vi "printFunc_preLabelPrint_wmg.vi"(7 "时间标识":timestamp format="%<%y/%m/%d>T", 8 "路径":path, 9 "Data in":string[](array[string]), 10 "input_str_PN":string="1", 11 "VISA resource name":refnum<visa-resource-name>="USB0::0x0A5F::0x00AB::JJL045601::RAW") -> (0 "exsit":bool, 3 "条码输出":string)   [LabVIEW 2011]
uses:
  <vilib>/Utility/file.llb/Read From Spreadsheet File (string).vi
  <vilib>/Utility/file.llb/Write To Spreadsheet File (string).vi
panel:
  # "0. P/N  luxshare\n1. Product Type *\n2. AWG\n3. Length\n4. SN\n5. Rev\n6. Custmer PN \n7. Vendor Number *\n8. Location *\n9. Label Title *"
  # "P/N  luxshare"
  # "Product Type *"
  # "AWG"
  # "Length"
  # "SN"
  # "Rev"
  # "Customer"
  # "Vender Num *"
  # "Location *"
  # "Label Title *"
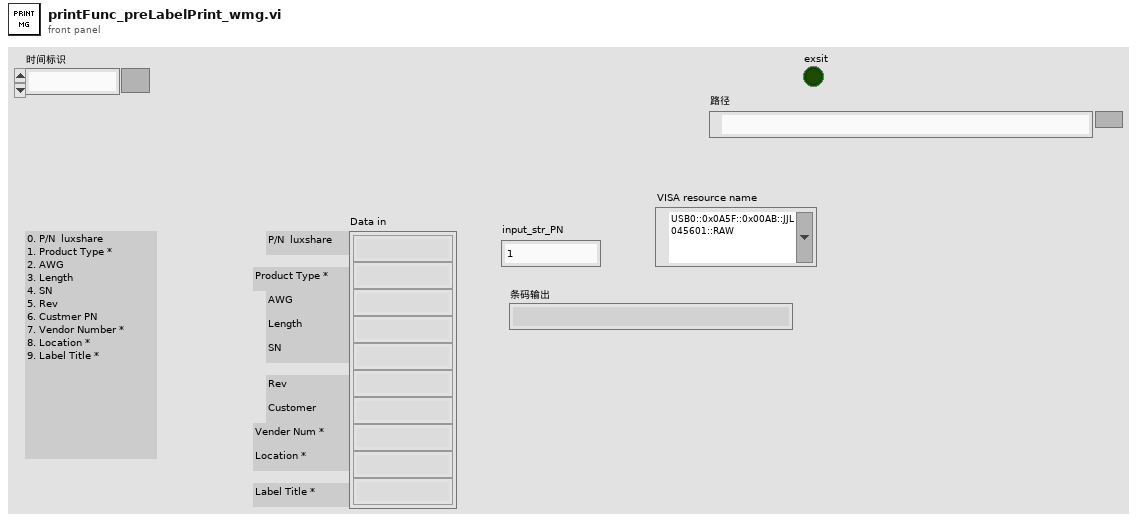
[diagram p1: front panel]
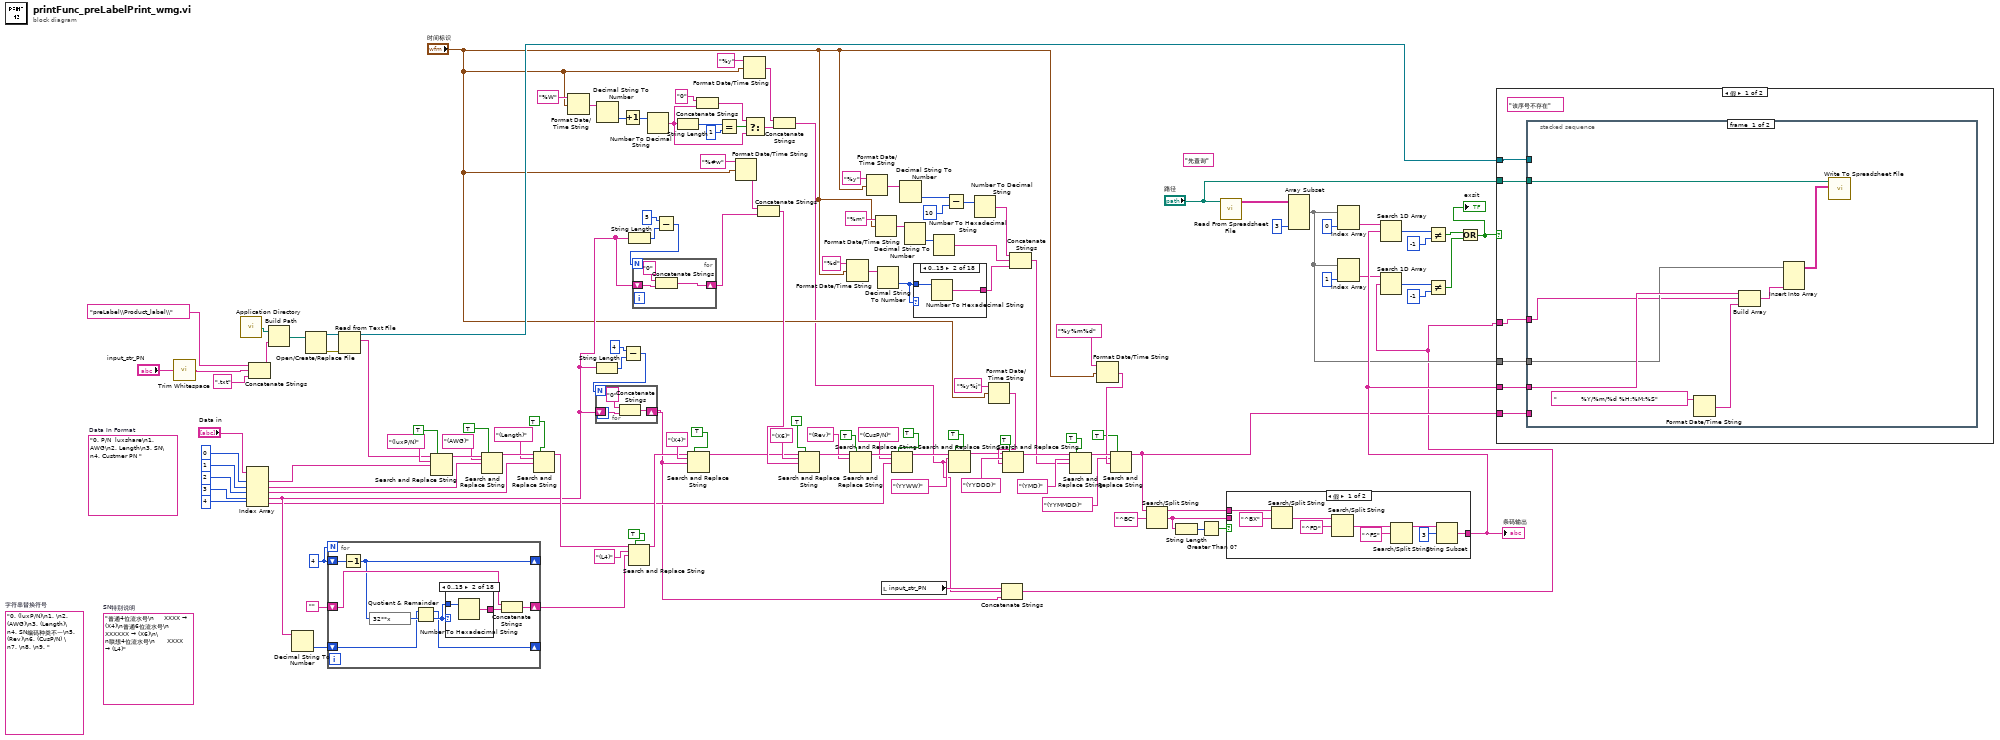
[diagram p0: block diagram]
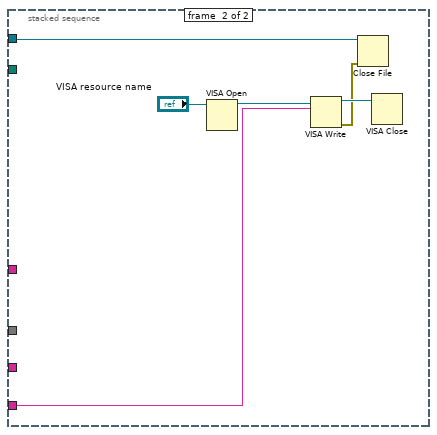
[diagram p2: hidden frame]
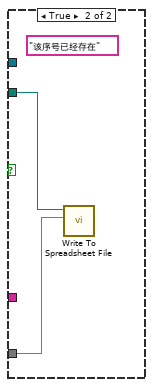
[diagram p3: hidden frame]
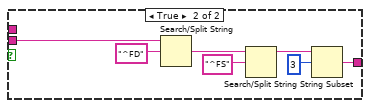
[diagram p4: hidden frame]
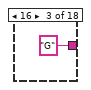
[diagram p6: hidden frame]
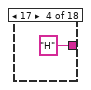
[diagram p7: hidden frame]
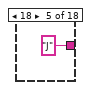
[diagram p8: hidden frame]
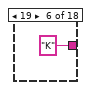
[diagram p9: hidden frame]
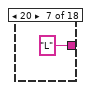
[diagram p10: hidden frame]
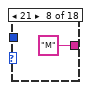
[diagram p11: hidden frame]
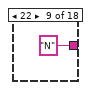
[diagram p12: hidden frame]
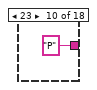
[diagram p13: hidden frame]
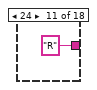
[diagram p14: hidden frame]
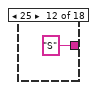
[diagram p15: hidden frame]
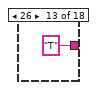
[diagram p16: hidden frame]
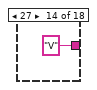
[diagram p17: hidden frame]
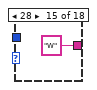
[diagram p18: hidden frame]
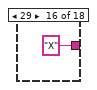
[diagram p19: hidden frame]
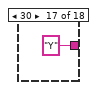
[diagram p20: hidden frame]
diagram:
  (unwired) "先查询"
  (unwired) "普通4位流水号\n     XXXX → (X4)\n普通6位流水号\n     XXXXXX → (X6)\n\n联想4位流水号\n      XXXX → (L4)"  # SN特别说明
  w68 = 4
  (unwired) "0. (luxP/N)\n1. \n2. (AWG)\n3. (Length)\n4. SN编码种类不一\n5. (Rev)\n6. (CusP/N) \n7. \n8. \n9. "  # 字符串替换符号
  (unwired) "0. P/N  luxshare\n1. AWG\n2. Length\n3. SN\n4. Custmer PN "  # Data In Format
  n1 = call <vilib>:"Trim Whitespace.vi"("string"="input_str_PN") -> ("trimmed string"=w60:string)  [unwired: 1 in]
  n2 = call <vilib>:"Application Directory.vi"() -> ("Application Directory"=w75:path)
  n3 = Index Array(array="Data in", index #1=0 ("索引"), index #2=1 ("索引"), index #3=2 ("索引"), index #4=3 ("索引"), index #5=4 ("索引")) -> (element #1=w116:string, element #2=w30:string, element #3=w28:string, element #4=w29:string, element #5=w27:string)
  n4 = Concatenate Strings("preLabel\\Product_label\\" ("名称或相对路径"), w60, ".txt" ("字符串")) -> (w74:string)
  n5 = Build Path(base path=w75, name or relative path=w74) -> (appended path=w71:path)
  n6 = Decimal String To Number(string=w29) -> (number=w67:i32)  [unwired: 2 in, 1 out]
  n7 = Open/Create/Replace File(file path (use dialog)=w71) -> (refnum out=w72:refnum<file>, error out=w73:errorcluster)  [unwired: 5 in, 1 out]
  n8 = for {
    N: w68 -> [_]
    shift-right: [w135] -> w65
    shift-left: "" -> [w136]
    shift-right: [w133] -> _
    shift-left: w68 -> [w134]
    shift-right: [w131] -> _
    shift-left: w67 -> [w132]
    n9 = Decrement(x=w134) -> (x-1=w133:i32)
    n10 = expression code="32**x"(w133) -> (w139:i32)
    n11 = Quotient & Remainder(x=w132, y=w139) -> (x-y*floor(x/y)=w131:i32, floor(x/y)=w138:i32)
    n12 = case shown="0..15" w138 {
      tunnel: w138 -> [_ w141 _ _ _ _ _ _ _ _ _ _ _ _ _ _ _ _]
      tunnel: [_ w140 "G" "H" "J" "K" "L" "M" "N" "P" "R" "S" "T" "V" "W" "X" "Y" "Z"] -> w137
      frame Default {
      }
      frame 0..15 {
        n13 = Number To Hexadecimal String(2:w141) -> (0:w140:string)  [unwired: 1 in]
      }
      frame 16 {
      }
      frame 17 {
      }
      frame 18 {
      }
      frame 19 {
      }
      frame 20 {
      }
      frame 21 {
      }
      frame 22 {
      }
      frame 23 {
      }
      frame 24 {
      }
      frame 25 {
      }
      frame 26 {
      }
      frame 27 {
      }
      frame 28 {
      }
      frame 29 {
      }
      frame 30 {
      }
      frame 31 {
      }
    }
    n14 = Concatenate Strings(w136, w137) -> (w135:string)
  }
  n15 = Read from Text File(file (use dialog)=w72, error in=w73) -> (refnum out=w17:refnum<file>, text=w70:string)  [unwired: 2 in, 2 out]
  n16 = Search and Replace String(replace all?=TRUE ("替换全部？(F)"), input string=w70, search string="(luxP/N)" ("搜索字符串"), replace string=w116) -> (result string=w115:string)  [unwired: 4 in, 3 out]
  n17 = Search and Replace String(replace all?=TRUE ("替换全部？(F)"), input string=w115, search string="(AWG)" ("搜索字符串"), replace string=w30) -> (result string=w114:string)  [unwired: 4 in, 3 out]
  n18 = Search and Replace String(replace all?=TRUE ("替换全部？(F)"), input string=w114, search string="(Length)" ("搜索字符串"), replace string=w28) -> (result string=w63:string)  [unwired: 4 in, 3 out]
  n19 = Format Date/Time String(time format string (%c)="%W" ("时间格式字符串(%c)"), seconds (now)="时间标识") -> (date/time string=w56:string)  [unwired: 1 in]
  n20 = String Length(string=w29) -> (length=w126:i32)
  n21 = Decimal String To Number(string=w56) -> (number=w55:i32)  [unwired: 2 in, 1 out]
  n22 = Increment(x=w55) -> (x+1=w54:i32)
  n23 = Subtract(x=4, y=w126) -> (x-y=w61:i32)
  n24 = for {
    N: w61 -> [_]
    shift-right: [w158] -> w3
    shift-left: w29 -> [w159]
    n25 = Concatenate Strings("0", w159) -> (w158:string)
  }
  n26 = Search and Replace String(replace all?=TRUE ("替换全部？(F)"), input string=w63, search string="(L4)" ("输入字符串"), replace string=w65) -> (result string=w62:string)  [unwired: 4 in, 3 out]
  n27 = String Length(string=w29) -> (length=w124:i32)
  n28 = Number To Decimal String(number=w54) -> (decimal integer string=w47:string)  [unwired: 1 in]
  n29 = Subtract(x=5, y=w124) -> (x-y=w125:i32)
  n30 = for {
    N: w125 -> [_]
    shift-right: [w161] -> w43
    shift-left: w29 -> [w162]
    n31 = Concatenate Strings("0", w162) -> (w161:string)
  }
  n32 = String Length(string=w47) -> (length=w52:i32)
  n33 = Search and Replace String(replace all?=TRUE ("替换全部？(F)"), input string=w62, search string="(X4)" ("搜索字符串"), replace string=w3) -> (result string=w5:string)  [unwired: 4 in, 3 out]
  n34 = Concatenate Strings("0" ("字符串"), w47) -> (w48:string)
  n35 = Equal?(x=w52, y=1) -> (x = y?=w50:bool)
  n36 = Format Date/Time String(time format string (%c)="%#w", seconds (now)="时间标识") -> (date/time string=w44:string)  [unwired: 1 in]
  n37 = Format Date/Time String(time format string (%c)="%y" ("时间格式字符串(%c)"), seconds (now)="时间标识") -> (date/time string=w53:string)  [unwired: 1 in]
  n38 = Select(t=w48, s=w50, f=w47) -> (s? t:f=w46:string)
  n39 = Concatenate Strings(w44, w43) -> (w42:string)
  n40 = Concatenate Strings(w53, w46) -> (w2:string)
  n41 = Search and Replace String(replace all?=TRUE ("替换全部？(F)"), input string=w5, search string="(X6)" ("搜索字符串"), replace string=w42) -> (result string=w111:string)  [unwired: 4 in, 3 out]
  n42 = Format Date/Time String(time format string (%c)="%d" ("时间格式字符串(%c)"), seconds (now)="时间标识") -> (date/time string=w88:string)  [unwired: 1 in]
  n43 = Search and Replace String(replace all?=TRUE ("替换全部？(F)"), input string=w111, search string="(Rev)" ("搜索字符串")) -> (result string=w109:string)  [unwired: 5 in, 3 out]
  n44 = Format Date/Time String(time format string (%c)="%y" ("时间格式字符串(%c)"), seconds (now)="时间标识") -> (date/time string=w86:string)  [unwired: 1 in]
  n45 = Format Date/Time String(time format string (%c)="%m" ("时间格式字符串(%c)"), seconds (now)="时间标识") -> (date/time string=w90:string)  [unwired: 1 in]
  n46 = Decimal String To Number(string=w88) -> (number=w81:i32)  [unwired: 2 in, 1 out]
  n47 = local read "input_str_PN"() -> (w7:string)
  n48 = Search and Replace String(replace all?=TRUE ("替换全部？(F)"), input string=w109, search string="(CusP/N)" ("搜索字符串"), replace string=w27) -> (result string=w100:string)  [unwired: 4 in, 3 out]
  n49 = Decimal String To Number(string=w86) -> (number=w84:i32)  [unwired: 2 in, 1 out]
  n50 = Decimal String To Number(string=w90) -> (number=w89:i32)  [unwired: 2 in, 1 out]
  n51 = case shown="0..15" w81 {
    tunnel: w81 -> [_ w165 _ _ _ _ _ _ _ _ _ _ _ _ _ _ _ _]
    tunnel: [_ w164 "G" "H" "J" "K" "L" "M" "N" "P" "R" "S" "T" "V" "W" "X" "Y" "Z"] -> w79
    frame Default {
    }
    frame 0..15 {
      n52 = Number To Hexadecimal String(2:w165) -> (0:w164:string)  [unwired: 1 in]
    }
    frame 16 {
    }
    frame 17 {
    }
    frame 18 {
    }
    frame 19 {
    }
    frame 20 {
    }
    frame 21 {
    }
    frame 22 {
    }
    frame 23 {
    }
    frame 24 {
    }
    frame 25 {
    }
    frame 26 {
    }
    frame 27 {
    }
    frame 28 {
    }
    frame 29 {
    }
    frame 30 {
    }
    frame 31 {
    }
  }
  n53 = Number To Hexadecimal String(2:w89) -> (0:w80:string)  [unwired: 1 in]
  n54 = Subtract(x=w84, y=10) -> (x-y=w83:i32)
  n55 = Search and Replace String(replace all?=TRUE ("替换全部？(F)"), input string=w100, search string="(YYWW)" ("搜索字符串"), replace string=w2) -> (result string=w6:string)  [unwired: 4 in, 3 out]
  n56 = Number To Decimal String(number=w83) -> (decimal integer string=w82:string)  [unwired: 1 in]
  n57 = Format Date/Time String(time format string (%c)="%y%j" ("时间格式字符串(%c)"), seconds (now)="时间标识") -> (date/time string=w59:string)  [unwired: 1 in]
  n58 = Concatenate Strings(w7, w2, w3) -> (w4:string)
  n59 = Search and Replace String(replace all?=TRUE ("替换全部？(F)"), input string=w6, search string="(YYDDD)" ("搜索字符串"), replace string=w59) -> (result string=w94:string)  [unwired: 4 in, 3 out]
  n60 = Concatenate Strings(w82, w80, w79) -> (w78:string)
  n61 = Search and Replace String(replace all?=TRUE ("替换全部？(F)"), input string=w94, search string="(YMD)" ("搜索字符串"), replace string=w78) -> (result string=w35:string)  [unwired: 4 in, 3 out]
  n62 = Format Date/Time String(time format string (%c)="%y%m%d" ("时间格式字符串(%c)"), seconds (now)="时间标识") -> (date/time string=w33:string)  [unwired: 1 in]
  n63 = Search and Replace String(replace all?=TRUE ("替换全部？(F)"), input string=w35, search string="(YYMMDD)" ("搜索字符串"), replace string=w33) -> (result string=w16:string)  [unwired: 4 in, 3 out]
  n64 = Search/Split String(string=w16, search string/char (-)="^BC" ("搜索字符串/字符(-)")) -> (substring before match=w38:string, match + rest of string=w37:string)  [unwired: 1 in, 1 out]
  n65 = String Length(string=w37) -> (length=w40:i32)
  n66 = Greater Than 0?(x=w40) -> (x > 0?=w39:bool)
  n67 = call-poly <vilib>:"Read From Spreadsheet File.vi"("file path (dialog if empty)"="路径") -> ("all rows"=w25:string[][])  [unwired: 6 in, 4 out]
  n68 = case shown="假" w39 {
    tunnel: w38 -> [w189 _]
    tunnel: w37 -> [_ w192]
    tunnel: [w182 w191] -> w19
    frame False {
      n69 = Search/Split String(string=w189, search string/char (-)="^BX" ("搜索字符串/字符(-)")) -> (match + rest of string=w183:string)  [unwired: 1 in, 2 out]
      n70 = Search/Split String(string=w183, search string/char (-)="^FD" ("搜索字符串/字符(-)")) -> (match + rest of string=w186:string)  [unwired: 1 in, 2 out]
      n71 = Search/Split String(string=w186, search string/char (-)="^FS" ("搜索字符串/字符(-)")) -> (substring before match=w185:string)  [unwired: 1 in, 2 out]
      n72 = String Subset(string=w185, offset (0)=3 ("偏移量(0)")) -> (substring=w182:string)  [unwired: 1 in]
    }
    frame True {
      n73 = Search/Split String(string=w192, search string/char (-)="^FD" ("搜索字符串/字符(-)")) -> (match + rest of string=w195:string)  [unwired: 1 in, 2 out]
      n74 = Search/Split String(string=w195, search string/char (-)="^FS" ("搜索字符串/字符(-)")) -> (substring before match=w194:string)  [unwired: 1 in, 2 out]
      n75 = String Subset(string=w194, offset (0)=3 ("偏移量(0)")) -> (substring=w191:string)  [unwired: 1 in]
    }
  }
  "条码输出" <- w19
  n76 = Array Subset(array=w25, length (col)=3 ("长度")) -> (w14:string[][])  [unwired: 3 in]
  n77 = Index Array(array=w14, index (col)=0 ("禁用的索引 (列)")) -> (element=w22:string[])  [unwired: 1 in]
  n78 = Index Array(array=w14, index (col)=1 ("禁用的索引 (列)")) -> (element=w10:string[])  [unwired: 1 in]
  n79 = Search 1D Array(1D array=w22, element=w19) -> (index of element=w21:i32)  [unwired: 1 in]
  n80 = Search 1D Array(1D array=w10, element=w4) -> (index of element=w11:i32)  [unwired: 1 in]
  n81 = Not Equal?(x=w21, y=-1) -> (x != y?=w9:bool)
  n82 = Not Equal?(x=w11, y=-1) -> (x != y?=w8:bool)
  n83 = Or(x=w9, y=w8) -> (x .or. y?=w1:bool)
  "exsit" <- w1
  n84 = case shown="假" w1 {
    tunnel: w19 -> [w203 _]
    tunnel: w14 -> [w202 w219]
    tunnel: "路径" -> [w201 w218]
    tunnel: w17 -> [w200 _]
    tunnel: w16 -> [w199 _]
    tunnel: w4 -> [w198 _]
    frame False {
      (unwired) "该序号不存在"
      n85 = stacked-sequence {
        tunnel: w203 -> [w210 _]
        tunnel: w202 -> [w209 _]
        tunnel: w201 -> [w207 _]
        tunnel: w200 -> [_ w213]
        tunnel: w199 -> [_ w212]
        tunnel: w198 -> [w204 _]
        frame #0 {
          n86 = Format Date/Time String(time format string (%c)="            %Y/%m/%d %H:%M:%S" ("时间格式字符串(%c)")) -> (date/time string=w205:string)  [unwired: 2 in]
          n87 = Build Array(w210, w204, w205) -> (w208:string[])
          n88 = Insert Into Array(array=w209, new element=w208) -> (w206:string[][])  [unwired: 2 in]
          n89 = call-poly <vilib>:"Write To Spreadsheet File.vi"("2D data"=w206, "file path (dialog if empty)"=w207) -> ()  [unwired: 6 in, 1 out]
        }
        frame #1 {
          n90 = VISA Open(VISA resource name="VISA resource name") -> (VISA resource name=w217:refnum<visa-resource-name>)  [unwired: 4 in, 1 out]
          n91 = VISA Write(VISA resource name=w217, write buffer=w212) -> (VISA resource name out=w216:refnum<visa-resource-name>, error out=w215:errorcluster)  [unwired: 1 in, 1 out]
          n92 = Close File(refnum=w213, error in=w215) -> ()  [unwired: 2 out]
          n93 = VISA Close(VISA resource name=w216) -> ()  [unwired: 1 in, 1 out]
        }
      }
    }
    frame True {
      (unwired) "该序号已经存在"
      n94 = call-poly <vilib>:"Write To Spreadsheet File.vi"("2D data"=w219, "file path (dialog if empty)"=w218) -> ()  [unwired: 6 in, 1 out]
    }
  }
